vi "Do.vi"(8 "error in":errorcluster, 10 "Actor in":refnum<class "Actor.lvclass">, 11 "Change Flow Rate MSG":refnum<class "Change Setpoint MSG.lvclass">) -> (0 "error out":errorcluster, 2 "Actor out":refnum<class "Actor.lvclass">)   [LabVIEW 2015, in "Alicat Lib.lvlib" / "Change Setpoint MSG.lvclass"]
doc: "(<B>Filename</B>: Actor Framework.lvlib:Message.lvclass:Do.vi)\n\nDefines what a message does when it is received by an actor. Generally, a message instructs an actor to invoke one of its methods. By default, this method does nothing. A child class must override it to define behavior. Create a child class by using the Actor Framework Message Maker dialog box."
uses:
  Change Setpoint MSG.lvclass
  <vilib>/ActorFramework/Actor/Actor.lvclass
  <vilib>/MSR Consulting, LLC/DAQ Device/Device/Device.lvclass
  Alicat Device.lvclass
  <vilib>/MSR Consulting, LLC/DAQ Device/Device/Device.lvclass/Device.ctl
  Change Setpoint MSG.lvclass/Change Setpoint MSG.ctl
  <vilib>/MSR Consulting, LLC/DAQ Device/Device/Read Configurable Device.vi
  <vilib>/MSR Consulting, LLC/Configurable Device/Configurable Device.lvclass
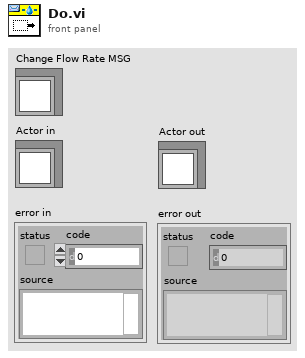
[diagram p1: front panel]
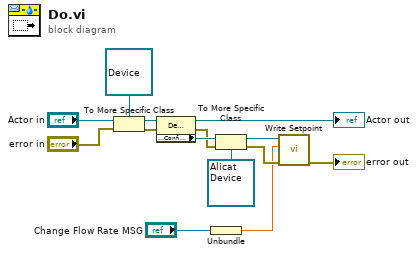
[diagram p0: block diagram]
diagram:
  n1 = To More Specific Class(target class=refnum<class "Device.lvclass"> refnum ("DAQ Device.lvlib:Device"), reference="Actor in", error in="error in") -> (specific class reference=w12:refnum<class "Device.lvclass">, error out=w8:errorcluster)
  n2 = property class="Device"(reference=w12, error in=w8) -> (reference out=→"Actor out":refnum<class "Device.lvclass">, error out=w7:errorcluster, "Accessors:Configurable Device"=w11:refnum<class "Configurable Device.lvclass">)
  n3 = Unbundle("Change Flow Rate MSG") -> (w1:dbl)
  n4 = To More Specific Class(target class=refnum<class "Alicat Device.lvclass"> refnum ("Alicat Device"), reference=w11, error in=w7) -> (specific class reference=w5:refnum<class "Alicat Device.lvclass">, error out=w4:errorcluster)
  n5 = call "Write Setpoint.vi"("error in"=w4, "Setpoint"=w1, "Alicat Device in"=w5) -> ("error out"=→"error out":errorcluster)  [unwired: 6 in, 2 out]
